vi "Create.vi"(8 "error in (no error)":errorcluster, 11 "File Type":T1) -> (0 "error out":errorcluster, 3 "Data out":refnum<class "Data.lvclass">)   [LabVIEW 2020, in "Data.lvclass"]
uses:
  Data.lvclass
  Typedefs/File Type--enum.ctl
  Data.DAT/Data.DAT.lvclass
  C:/user/phil/LV-to-ITX/src/Data/Data.lvclass
  Data.ITX/Data.ITX.lvclass
  Data.TDMS/Data.TDMS.lvclass
  Data.PG/Data.PG.lvclass
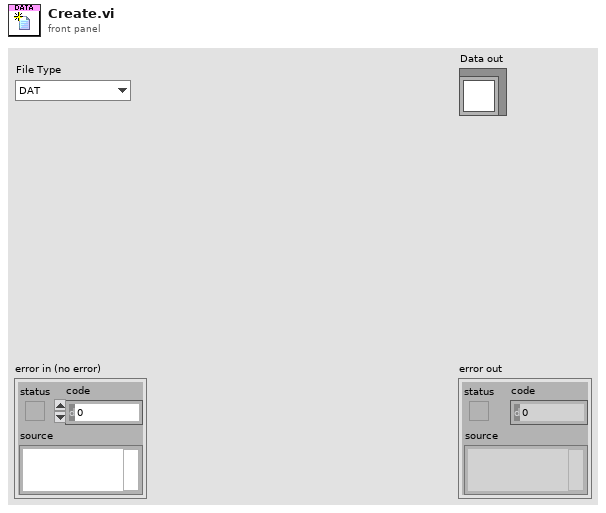
[diagram p1: front panel]
types:
  T1 = typedef "Data.lvclass/File Type--enum.ctl" = enum16{"DAT", "ITX", "TDMS", "VI", "PGSQL"}
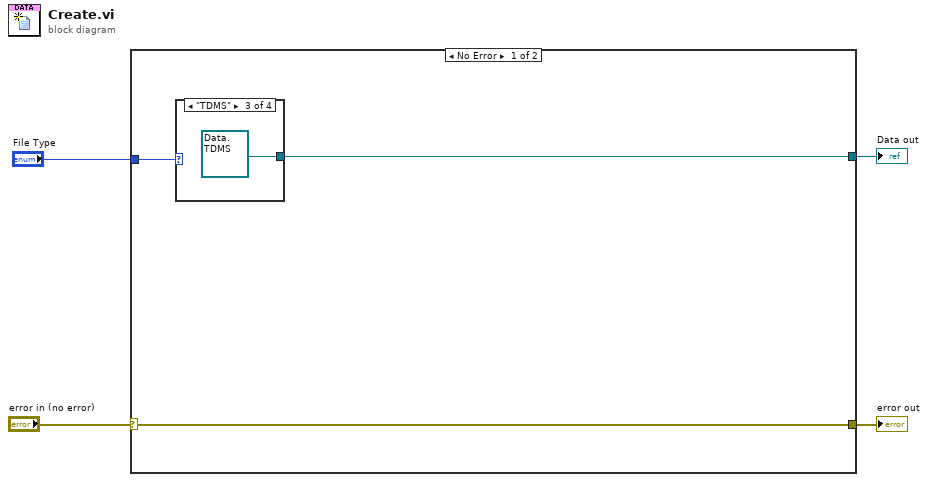
[diagram p0: block diagram]
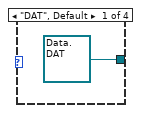
[diagram p2: hidden frame]
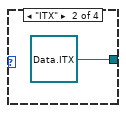
[diagram p3: hidden frame]
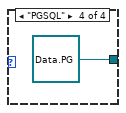
[diagram p4: hidden frame]
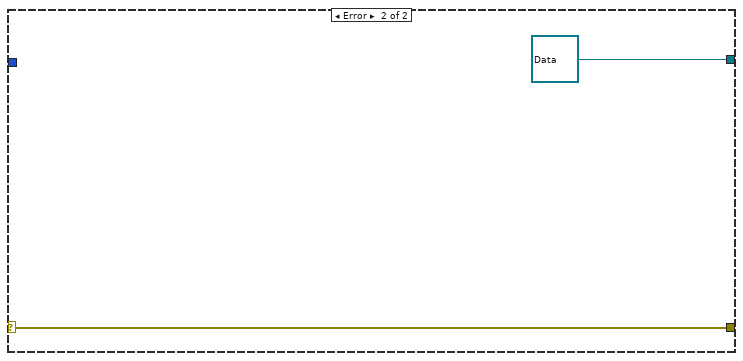
[diagram p5: hidden frame]
diagram:
  n1 = case shown="No Error" "error in (no error)" {
    selector: "error in (no error)" -> [w7 w13]
    tunnel: [w7 w13] -> w3
    tunnel: [w5 refnum<class "Data.lvclass"> refnum ("ITX")] -> w2
    tunnel: "File Type" -> [w6 _]
    frame No Error {
      n2 = case shown="\"TDMS\"" w6 {
        tunnel: [refnum<class "Data.DAT.lvclass"> refnum ("DAT.lvclass") refnum<class "Data.ITX.lvclass"> refnum ("ITX") refnum<class "Data.TDMS.lvclass"> refnum ("Data.TDMS.lvclass") refnum<class "Data.PG.lvclass"> refnum ("Data.PG.lvclass")] -> w5
        frame "DAT", Default {
        }
        frame "ITX" {
        }
        frame "TDMS" {
        }
        frame "PGSQL" {
        }
      }
    }
    frame Error {
    }
  }
  "error out" <- w3
  "Data out" <- w2
